vi "arrayenum.vi"(1 "Array In":enum16{"a", "b", "c", "d"}[](array[ring])) -> (0 "Array Out":enum16{"a", "b", "c", "d"}[](array[ring]))   [LabVIEW 2013]
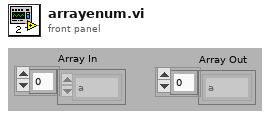
[diagram p1: front panel]
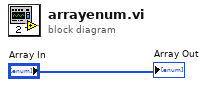
[diagram p0: block diagram]
diagram:
  "Array Out" <- "Array In"
